vi "Truncate 2D Array.vi"(3 "2D Array":sgl[][](array[numeric])) -> (0 "Header Index":i32[](array[numeric]), 1 "Truncated 2D Array":sgl[][](array[numeric]))   [LabVIEW 2016]
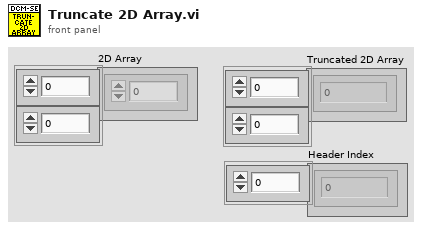
[diagram p1: front panel]
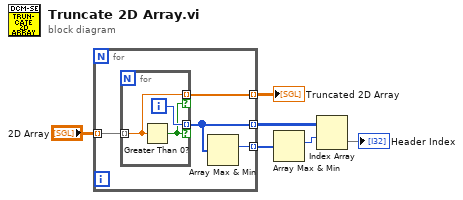
[diagram p0: block diagram]
diagram:
  n1 = for {
    tunnel: "2D Array" -> [w10] mode=indexing
    tunnel: [w9] -> w5 mode=indexing
    tunnel: [w8] -> w4 mode=indexing
    tunnel: [w7] -> w2 mode=indexing
    n2 = for {
      tunnel: [w13] -> w9 mode=indexing if=w11
      tunnel: w10 -> [w13] mode=indexing
      tunnel: [w12] -> w7 mode=indexing if=w11
      i -> [w12]
      n3 = Greater Than 0?(x=w13) -> (x > 0?=w11:bool)
    }
    n4 = Array Max & Min(array=w7) -> (max index (indices)=w8:i32)  [unwired: 3 out]
  }
  "Truncated 2D Array" <- w5
  n5 = Array Max & Min(array=w4) -> (max index (indices)=w3:i32)  [unwired: 3 out]
  n6 = Index Array(array=w2, index (row)=w3) -> (element=→"Header Index":i32[])  [unwired: 1 in]
